vi "8channels_LEEMAN_081413.vi"() -> ()   [LabVIEW 2012]
doc: "Cont(inuous) Acq(uire) & Chart (hw timed) demonstrates the hardware timed, non-buffered technique of data acquisition. The scan clock on the board controls acquisition timing. Acquired scans are read directly from the device's FIFO using AI Single Scan. \n\nThe acquisition is configured with no buffer, and the on-board scan clock started at the selected scan rate. In the first loop iteration, the newest (most recent) scan is read from the FIFO. In each subsequent loop iteration AI Single Scan is called to read the oldest scan from the FIFO. Then if a scan is missed because the acquisition does not keep up, an error message will be displayed, and the acquisition stopped. Each scan is plotted on the chart after it is read. \n\nA common reason to use non-buffered acquisition is that some kind of processing needs to be done for each data point. You will probably want to add more functions to the diagram to customize this VI for your application. The acquisition rate you can achieve depends on how much processing and display the VI must do. This VI calls a subVI named My Single-Scan Processing. Add whatever processing you need to this subVI, or replace it with one of your own. The data processing subVI also demonstrates how to use error clusters in your own subVIs, so they can be included in the error data flow chain.\n\nBefore running this VI, set the values of the controls on the front panel. Select Show Help Window from the Help menu to see a description of each control. If the values you select for all the controls are values you will usually use, select Make Current Values Default from the Operate menu and save the VI. Or, you may save individual control's default values by popping up on the control, selecting Data Operations, then selecting Make Current Value Default, and saving the VI."
uses:
  <vilib>/DAQmx/read.llb/DAQmx Read (Analog 2D DBL NChan NSamp).vi
  BiaxGlobals.vi
  <vilib>/DAQmx/create/channels.llb/DAQmx Create Channel (AI-Voltage-Basic).vi
  <vilib>/DAQmx/configure/timing.llb/DAQmx Timing (Sample Clock).vi
  <vilib>/DAQmx/miscellaneous.llb/DAQmx Fill In Error Info.vi
panel:
  out "element 11":string
  out "element 10":string
  out "element 9":string
  out "element 8":string
  out "element 7":string
  out "element 6":string
  out "element 5":string
  out "element 4":string
  out "element 3":string
  out "element 2":string
  out "element":string
  out "element":string
  out "Stress-strain-temp vs time (Voltage)":dbl[][](graph)
  out "Array 13":i32[][](array[numeric])
  out "Array 12":i32[][](array[numeric])
  out "AUX8 (ch11)":dbl format="%.4f"
  out "AUX7 (ch10)":dbl format="%.4f"
  out "Array 11":i32[][](array[numeric])
  out "Array 10":i32[][](array[numeric])
  out "AUX6 (ch9)":dbl format="%.4f"
  out "AUX5 (ch8)":dbl format="%.4f"
  out "Array 9":i32[][](array[numeric])
  out "Array 8":i32[][](array[numeric])
  out "Array 7":i32[][](array[numeric])
  out "Array 6":i32[][](array[numeric])
  out "Array 5":i32[][](array[numeric])
  out "Array 4":i32[][](array[numeric])
  out "Array 3":i32[][](array[numeric])
  out "Array 2":i32[][](array[numeric])
  out "Array":i32[][](array[numeric])
  out "AUX4 (ch7)":dbl format="%.4f"
  out "AUX3 (ch6)":dbl format="%.4f"
  out "AUX2 (ch5)":dbl format="%.4f"
  out "AUX1 (ch4)":dbl format="%.4f"
  out "10000":bool
  in  "10 kHz":bool
  out "Processor scan rate":i32
  out "Present sample number":i32
  in  "1 Hz":bool
  out "1":bool
  out "10":bool
  out "100":bool
  out "1000":bool
  in  "10 Hz":bool
  in  "100 Hz":bool
  in  "1000 Hz":bool
  out "Data Recording Rate":i32(slide) scale=1.0..10000.0
  out "Write interval":i32
  out "Write countdown":i32
  out "Time into data acq. (s)":i32
  out "Saved sample No.":i32
  out "Record rate (samp/s)":i32
  out "No. of scans in backlog":i32
  out "Vert LVDT (ch3)":dbl format="%.4f"
  out "Vert Load (ch2)":dbl format="%.4f"
  out "Hor Load (ch0)":dbl format="%.4f"
  out "Hor LVDT (ch1)":dbl format="%.4f"
  in  "stop":bool
  # "Input Signals (volts)"
  # "To File (32 bit)"
  # "S\nI\nG\nN\nA\nL\n\nV\nO\nL\nT\nA\nG\nE"
  # "Timestamp"
  # "Acquisition Statistics"
  # "Data Recording Info"
  # "Sample (point) Number"
  # "NOTE:  This instrument will write data (time channel then Channels 0-3) to a user defined filename.  The file is written in binary format without a header.  \n            The time channel is comprised of numbers indicating the data recording frequency (eg 1, 10, 100, 1000, 10000  samples per second)."
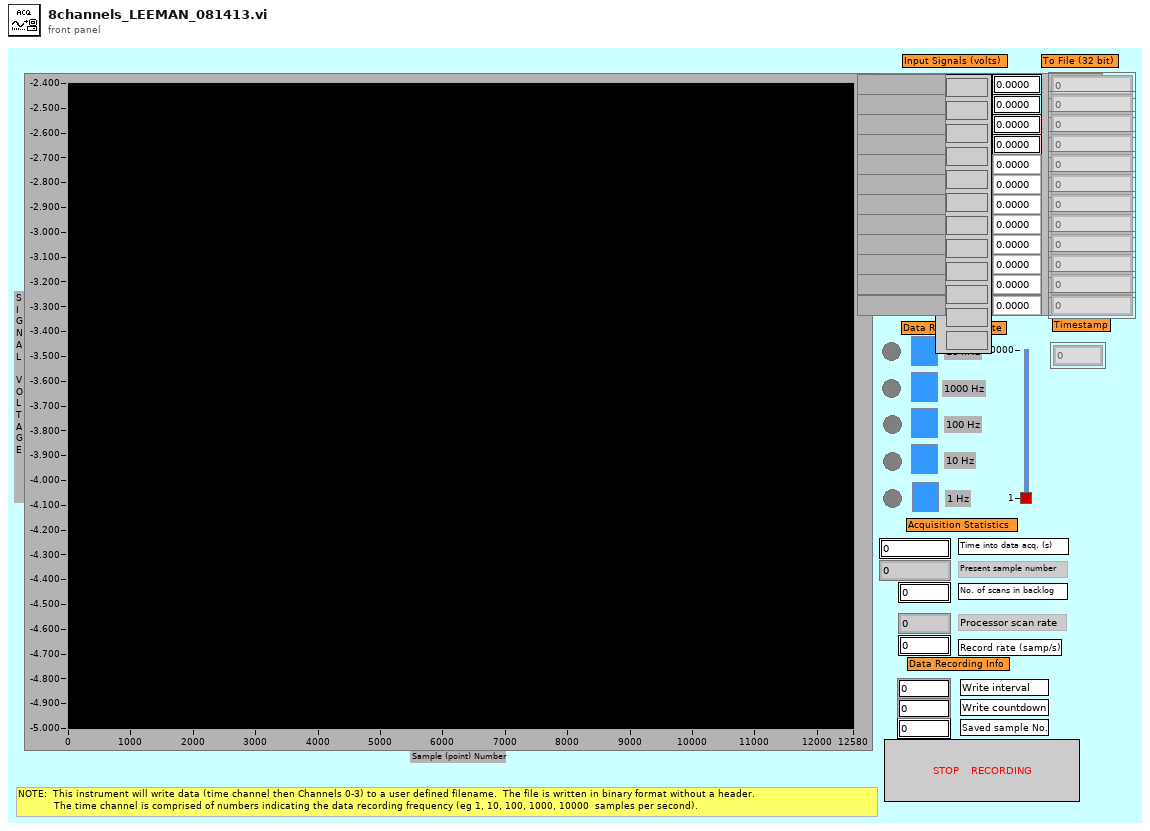
[diagram p1: front panel]
types:
  T1 = enum16{"big-endian, network order", "native, host order", "little-endian"}
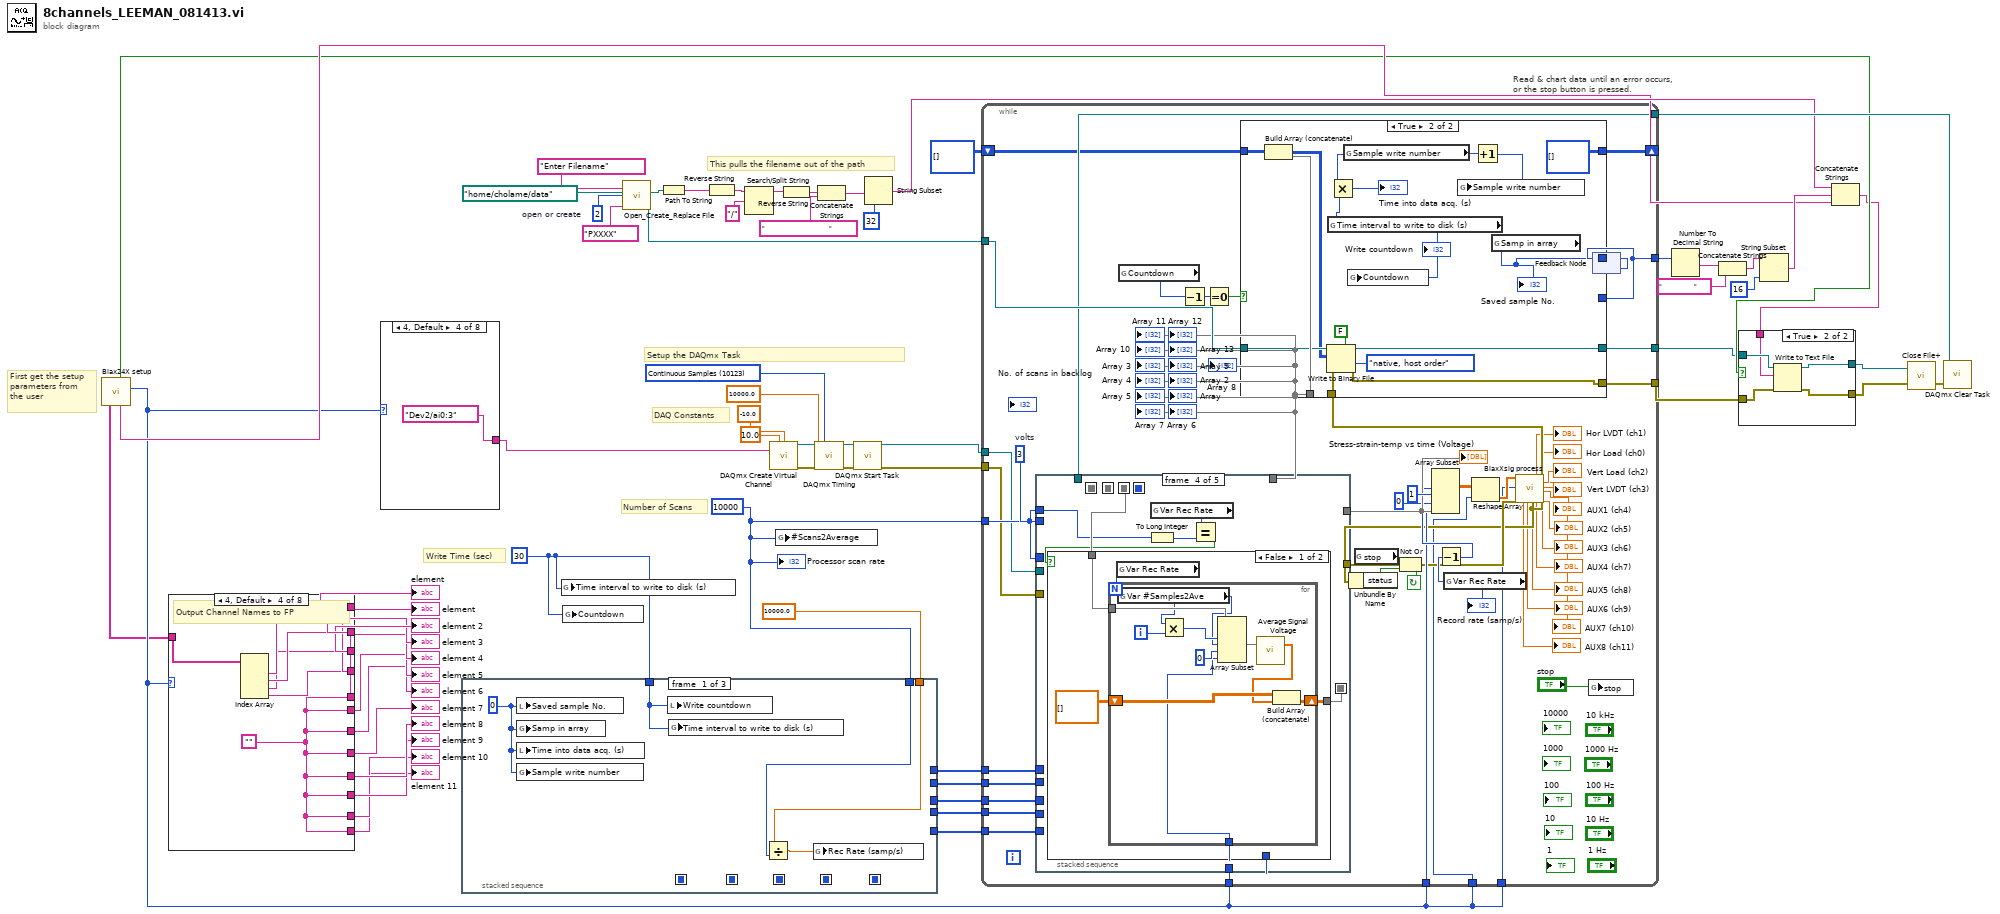
[diagram p0: block diagram]
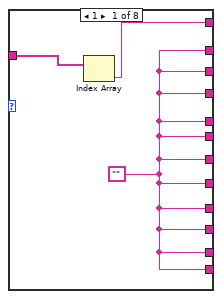
[diagram p2: hidden frame]
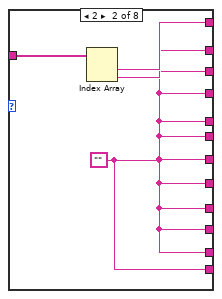
[diagram p3: hidden frame]
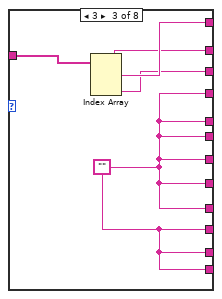
[diagram p4: hidden frame]
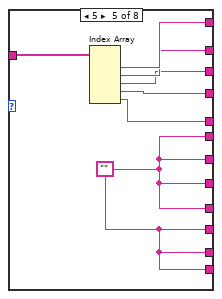
[diagram p5: hidden frame]
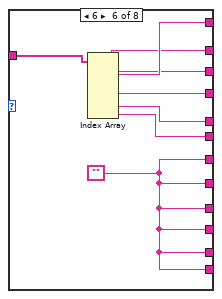
[diagram p6: hidden frame]
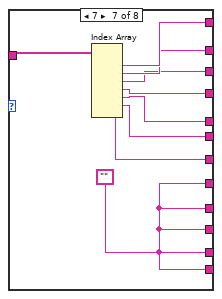
[diagram p7: hidden frame]
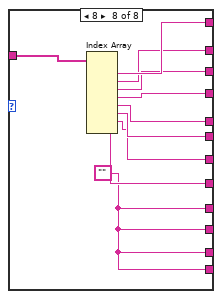
[diagram p8: hidden frame]
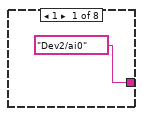
[diagram p10: hidden frame]
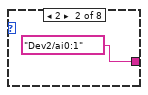
[diagram p11: hidden frame]
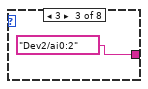
[diagram p12: hidden frame]
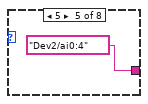
[diagram p13: hidden frame]
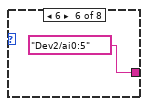
[diagram p14: hidden frame]
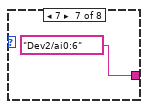
[diagram p15: hidden frame]
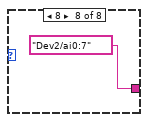
[diagram p16: hidden frame]
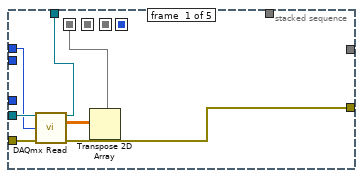
[diagram p17: hidden frame]
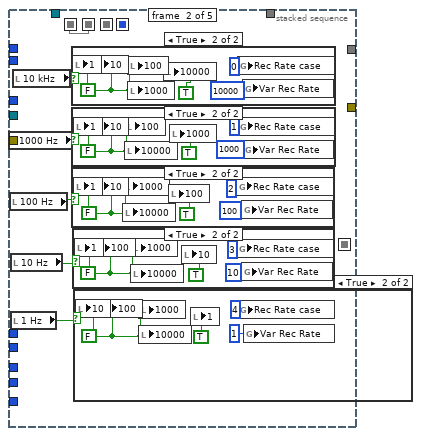
[diagram p18: hidden frame]
diagram:
  w6 = 10000 ("Number of scans")
  w7 = 30 ("Write time int (s)")
  w48 = 10123 items=["Finite Samples"=10178, "Continuous Samples"=10123, "Hardware Timed Single Point"=12522] ("sample mode")
  w64 = 2  # open or create
  # "Number of Scans"
  # "Write Time (sec)"
  # "First get the setup\nparameters from\nthe user"
  # "Setup the DAQmx Task"
  # "DAQ Constants"
  # "This pulls the filename out of the path"
  n1 = call "Biax24X setup.vi"() -> ("Footer String"=w29:string, "Number of Channels"=w22:i32, "ASCII footer 2"=w28:bool, "Channel Names"=w21:string[])  [unwired: 1 in, 4 out]
  n2 = case shown="4, Default" w22 {
    tunnel: w21 -> [w66 w70 w75 w81 w88 w96 w105 w116]
    tunnel: [w65 w71 w76 w82 w89 w97 w106 w115] -> w20
    tunnel: [w67 w69 w74 w80 w87 w95 w104 w114] -> w19
    tunnel: [w67 w68 w73 w79 w86 w94 w103 w113] -> w18
    tunnel: [w67 w68 w72 w78 w85 w93 w102 w112] -> w17
    tunnel: [w67 w68 w72 w77 w84 w92 w101 w111] -> w16
    tunnel: [w67 w68 w72 w77 w83 w91 w100 w110] -> w15
    tunnel: [w67 w68 w72 w77 w83 w90 w99 w109] -> w14
    tunnel: [w67 w68 w72 w77 w83 w90 w98 w108] -> w13
    tunnel: [w67 w68 w72 w77 w83 w90 w98 w107] -> w12
    tunnel: [w67 w68 w72 w77 w83 w90 w98 w107] -> w11
    tunnel: [w67 w68 w72 w77 w83 w90 w98 w107] -> w10
    tunnel: [w67 w68 w72 w77 w83 w90 w98 w107] -> w9
    frame 1 {
      w67 = ""
      n3 = Index Array(array=w66) -> (element=w65:string)  [unwired: 1 in]
    }
    frame 2 {
      w68 = ""
      n4 = Index Array(array=w70) -> (element #1=w71:string, element #2=w69:string)  [unwired: 2 in]
    }
    frame 3 {
      w72 = ""
      n5 = Index Array(array=w75) -> (element #1=w76:string, element #2=w74:string, element #3=w73:string)  [unwired: 3 in]
    }
    frame 4, Default {
      w77 = ""
      # "Output Channel Names to FP"
      n6 = Index Array(array=w81) -> (element #1=w82:string, element #2=w80:string, element #3=w79:string, element #4=w78:string)  [unwired: 4 in]
    }
    frame 5 {
      w83 = ""
      n7 = Index Array(array=w88) -> (element #1=w89:string, element #2=w87:string, element #3=w86:string, element #4=w85:string, element #5=w84:string)  [unwired: 5 in]
    }
    frame 6 {
      w90 = ""
      n8 = Index Array(array=w96) -> (element #1=w97:string, element #2=w95:string, element #3=w94:string, element #4=w93:string, element #5=w92:string, element #6=w91:string)  [unwired: 6 in]
    }
    frame 7 {
      w98 = ""
      n9 = Index Array(array=w105) -> (element #1=w106:string, element #2=w104:string, element #3=w103:string, element #4=w102:string, element #5=w101:string, element #6=w100:string, element #7=w99:string)  [unwired: 7 in]
    }
    frame 8 {
      w107 = ""
      n10 = Index Array(array=w116) -> (element #1=w115:string, element #2=w114:string, element #3=w113:string, element #4=w112:string, element #5=w111:string, element #6=w110:string, element #7=w109:string, element #8=w108:string)  [unwired: 8 in]
    }
  }
  "element" <- w20
  "element" <- w19
  "element 2" <- w18
  "element 3" <- w17
  "element 4" <- w16
  "element 5" <- w15
  "element 6" <- w14
  "element 7" <- w13
  "element 8" <- w12
  "element 9" <- w11
  "element 10" <- w10
  "element 11" <- w9
  n11 = case shown="4, Default" w22 {
    tunnel: [tag "Dev2/ai0" ("physical channels") tag "Dev2/ai0:1" ("physical channels") tag "Dev2/ai0:2" ("physical channels") tag "Dev2/ai0:3" ("physical channels") tag "Dev2/ai0:4" ("physical channels") tag "Dev2/ai0:5" ("physical channels") tag "Dev2/ai0:6" ("physical channels") tag "Dev2/ai0:7" ("physical channels")] -> w37
    frame 1 {
    }
    frame 2 {
    }
    frame 3 {
    }
    frame 4, Default {
    }
    frame 5 {
    }
    frame 6 {
    }
    frame 7 {
    }
    frame 8 {
    }
  }
  n12 = stacked-sequence {
    seq-local: [_ w145 _] -> [_ _ w158]
    seq-local: [_ w142 _] -> [_ _ w155]
    seq-local: [_ w137 _] -> [_ _ w157]
    seq-local: [_ w136 _] -> [_ _ w156]
    seq-local: [_ w131 _] -> [_ _ w154]
    tunnel: w7 -> [w126 _ _]
    tunnel: w6 -> [w129 _ _]
    tunnel: sgl 10000.0 ("actual scan rate") -> [w127 _ _]
    tunnel: [_ _ w158] -> w5
    tunnel: [_ _ w155] -> w4
    tunnel: [_ _ w157] -> w3
    tunnel: [_ _ w156] -> w2
    tunnel: [_ _ w154] -> w1
    frame #0 {
      w125 = i16 0
      n13 = local write "Saved sample No."(w125) -> ()
      n14 = global write "BiaxGlobals.vi" "Samp in array"(w125) -> ()
      n15 = local write "Time into data acq. (s)"(w125) -> ()
      n16 = global write "BiaxGlobals.vi" "Sample write number"(w125) -> ()
      n17 = local write "Write countdown"(w126) -> ()
      n18 = global write "BiaxGlobals.vi" "Time interval to write to disk (s)"(w126) -> ()
      n19 = Divide(x=w127, y=w129) -> (x/y=w128:sgl)
      n20 = global write "BiaxGlobals.vi" "Rec Rate (samp/s)"(w128) -> ()
    }
    frame #1 {
      n21 = local write "1"(TRUE) -> ()
      n22 = local write "10"(FALSE) -> ()
      n23 = local write "100"(FALSE) -> ()
      n24 = local write "1000"(FALSE) -> ()
      n25 = local write "10000"(FALSE) -> ()
      n26 = global read "BiaxGlobals.vi" "Time interval to write to disk (s)"() -> (→"Write interval":i32)
      n27 = global write "BiaxGlobals.vi" "Rec Rate case"(4) -> ()
      n28 = Initialize Array(i16 1, 10000) -> (w145:i16[])
      n29 = Initialize Array(i16 10, 1000) -> (w142:i16[])
      n30 = Initialize Array(i16 100, 100) -> (w137:i16[])
      n31 = Initialize Array(i16 1000, 10) -> (w136:i16[])
      n32 = Initialize Array(i16 10000, 1) -> (w131:i16[])
      n33 = global write "BiaxGlobals.vi" "Accum Time"(0) -> ()
      n34 = global write "BiaxGlobals.vi" "Var Rec Rate"(1) -> ()
    }
    frame #2 {
    }
  }
  n35 = global write "BiaxGlobals.vi" "Time interval to write to disk (s)"(w7) -> ()
  n36 = global write "BiaxGlobals.vi" "Countdown"(w7) -> ()
  n37 = call <vilib>:"Open_Create_Replace File.vi"("default name"="PXXXX", "prompt"="Enter Filename", "function (open:0)"=w64, "start path  (Not A Path)"=path "/home/cholame/data") -> ("new file path"=w59:path, "refnum"=w61:refnum<file>)  [unwired: 4 in, 2 out]
  n38 = Path To String(path=w59) -> (string=w56:string)
  n39 = Reverse String(1:w56) -> (0:w57:string)
  n40 = Search/Split String(string=w57, search string/char (-)="/") -> (substring before match=w55:string)  [unwired: 1 in, 2 out]
  n41 = call-poly <vilib>:"DAQmx Create Virtual Channel.vi"("maximum value"=10.0, "minimum value"=-10.0, "physical channels"=w37) -> ("task out"=w50:refnum<k21>, "error out"=w49:errorcluster)  [unwired: 11 in]
  n42 = global write "BiaxGlobals.vi" "#Scans2Average"(w6) -> ()
  n43 = Reverse String(1:w55) -> (0:w51:string)
  n44 = call-poly <vilib>:"DAQmx Timing.vi"("task/channels in"=w50, "sample mode"=w48, "rate"=10000.0, "error in"=w49) -> ("task out"=w47:refnum<k21>, "error out"=w46:errorcluster)  [unwired: 10 in]
  n45 = Concatenate Strings(w51, "                                ") -> (w53:string)
  n46 = call <vilib>:"DAQmx Start Task.vi"("task/channels in"=w47, "error in"=w46) -> ("task out"=w43:refnum<k21>, "error out"=w44:errorcluster)  [unwired: 12 in]
  n47 = String Subset(string=w53, length (rest)=32 ("length (rest)")) -> (substring=w30:string)  [unwired: 1 in]
  n48 = while "Read & chart data until an error occurs,\nor the stop button is pressed." {
    shift-left: i16[][] [] -> [w171]
    shift-right: [w205] -> _
    tunnel: w6 -> [w191]
    tunnel: [w206] -> w24
    tunnel: [w207] -> w27
    tunnel: w61 -> [w208]
    tunnel: w22 -> [w188]
    tunnel: w22 -> [w174]
    tunnel: w22 -> [w187]
    tunnel: w22 -> [w175]
    tunnel: w44 -> [w167]
    tunnel: w43 -> [w166]
    tunnel: [w199] -> w42
    tunnel: [w164] -> w36
    tunnel: w5 -> [w163]
    tunnel: w4 -> [w162]
    tunnel: w3 -> [w161]
    tunnel: w2 -> [w160]
    tunnel: w1 -> [w159]
    stop <- w204 continue-if-true
    w198 = 3  # volts
    n49 = stacked-sequence {
      seq-local: [w209 _ _ _ _] -> [_ w218 _ _ _]
      seq-local: [_ w218 _ _ _] -> [_ _ w244 _ _]
      seq-local: [_ _ w244 _ _] -> [_ _ _ w268 _]
      seq-local: [_ _ w243 _ _] -> [_ _ _ _ w294]
      seq-local: [_ _ _ w265 _] -> [_ _ _ _ w290]
      tunnel: [w215 _ _ _ _] -> w199
      tunnel: w198 -> [_ _ _ _ _]
      tunnel: w191 -> [w211 _ _ w267 _]
      tunnel: [w214 _ _ _ _] -> w185
      tunnel: [_ _ _ _ w290] -> w195
      tunnel: w191 -> [_ _ _ _ w293]
      tunnel: w163 -> [_ _ w254 _ _]
      tunnel: w162 -> [_ _ w253 _ _]
      tunnel: w161 -> [_ _ w252 _ _]
      tunnel: w160 -> [_ _ w251 _ _]
      tunnel: [_ _ _ _ w291] -> w168
      tunnel: w159 -> [_ _ w242 _ _]
      tunnel: w187 -> [_ _ _ w263 _]
      tunnel: w167 -> [w213 _ _ _ _]
      tunnel: w166 -> [w212 _ _ _ _]
      frame #0 {
        n50 = call-poly <vilib>:"DAQmx Read.vi"("task/channels in"=w212, "number of samples per channel"=w211, "error in"=w213) -> ("task out"=w215:refnum<k21>, "data"=w210:dbl[][], "error out"=w214:errorcluster)  [unwired: 10 in]
        n51 = Transpose 2D Array(2D array=w210) -> (transposed array=w209:dbl[][])
      }
      frame #1 {
        n52 = local read "1000 Hz"() -> (w221:bool)
        n53 = local read "100 Hz"() -> (w220:bool)
        n54 = local read "10 Hz"() -> (w219:bool)
        n55 = local read "1 Hz"() -> (w217:bool)
        n56 = local read "10 kHz"() -> (w216:bool)
        n57 = case shown="True" w216 {
          frame False {
          }
          frame True {
            w222 = FALSE
            n58 = local write "1"(w222) -> ()
            n59 = local write "10"(w222) -> ()
            n60 = local write "100"(w222) -> ()
            n61 = local write "1000"(w222) -> ()
            n62 = local write "10000"(TRUE ("10x")) -> ()
            n63 = global write "BiaxGlobals.vi" "Rec Rate case"(0) -> ()
            n64 = global write "BiaxGlobals.vi" "Var Rec Rate"(10000) -> ()
          }
        }
        n65 = case shown="True" w221 {
          frame False {
          }
          frame True {
            w238 = FALSE
            n66 = local write "1"(w238) -> ()
            n67 = local write "10"(w238) -> ()
            n68 = local write "100"(w238) -> ()
            n69 = local write "10000"(w238) -> ()
            n70 = local write "1000"(TRUE ("10x")) -> ()
            n71 = global write "BiaxGlobals.vi" "Rec Rate case"(1) -> ()
            n72 = global write "BiaxGlobals.vi" "Var Rec Rate"(1000) -> ()
          }
        }
        n73 = case shown="True" w220 {
          frame False {
          }
          frame True {
            w234 = FALSE
            n74 = local write "1"(w234) -> ()
            n75 = local write "10"(w234) -> ()
            n76 = local write "1000"(w234) -> ()
            n77 = local write "10000"(w234) -> ()
            n78 = local write "100"(TRUE ("1x")) -> ()
            n79 = global write "BiaxGlobals.vi" "Rec Rate case"(2) -> ()
            n80 = global write "BiaxGlobals.vi" "Var Rec Rate"(100) -> ()
          }
        }
        n81 = case shown="True" w219 {
          frame False {
          }
          frame True {
            w230 = FALSE
            n82 = local write "1"(w230) -> ()
            n83 = local write "100"(w230) -> ()
            n84 = local write "1000"(w230) -> ()
            n85 = local write "10000"(w230) -> ()
            n86 = local write "10"(TRUE ("0.1x")) -> ()
            n87 = global write "BiaxGlobals.vi" "Rec Rate case"(3) -> ()
            n88 = global write "BiaxGlobals.vi" "Var Rec Rate"(10) -> ()
          }
        }
        n89 = case shown="True" w217 {
          frame False {
          }
          frame True {
            w226 = FALSE
            n90 = local write "10"(w226) -> ()
            n91 = local write "100"(w226) -> ()
            n92 = local write "1000"(w226) -> ()
            n93 = local write "10000"(w226) -> ()
            n94 = local write "1"(TRUE) -> ()
            n95 = global write "BiaxGlobals.vi" "Rec Rate case"(4) -> ()
            n96 = global write "BiaxGlobals.vi" "Var Rec Rate"(1) -> ()
          }
        }
      }
      frame #2 {
        n97 = global read "BiaxGlobals.vi" "Rec Rate case"() -> (w250:i32)
        n98 = case shown="3" w250 {
          tunnel: w254 -> [w258 _ _ _ _]
          tunnel: [w258 w259 w260 w261 w262] -> w243
          tunnel: w253 -> [_ w259 _ _ _]
          tunnel: w252 -> [_ _ w260 _ _]
          tunnel: w251 -> [_ _ _ w261 _]
          tunnel: w242 -> [_ _ _ _ w262]
          frame ..0 {
          }
          frame 1 {
          }
          frame 2 {
          }
          frame 3 {
          }
          frame 4.. {
          }
        }
        n99 = Array Size(array=w243) -> (size(s)=w247:i32)
        n100 = global read "BiaxGlobals.vi" "Countdown"() -> (w246:i32)
        n101 = global read "BiaxGlobals.vi" "Samp in array"() -> (w249:i32)
        n102 = Add(x=w249, y=w247) -> (x+y=w248:i32)
        "Present sample number" <- w248
        n103 = global read "BiaxGlobals.vi" "Var Rec Rate"() -> (w256:i32)
        "Data Recording Rate" <- w256
        n104 = global write "BiaxGlobals.vi" "Samp in array"(w248) -> ()
        n105 = global read "BiaxGlobals.vi" "#Scans2Average"() -> (w257:i16)
        n106 = Divide(x=w257, y=w256) -> (x/y=w255:dbl)
        n107 = Decrement(x=w246) -> (x-1=w245:i32)
        n108 = global write "BiaxGlobals.vi" "Var #Samples2Ave"(w255) -> ()
        n109 = local write "Write countdown"(w245) -> ()
      }
      frame #3 {
        n110 = To Long Integer(number=w267) -> (32bit integer=w266:i32)
        n111 = global read "BiaxGlobals.vi" "Var Rec Rate"() -> (w269:i32)
        n112 = Equal?(x=w269, y=w266) -> (x = y?=w264:bool)
        n113 = case shown="False" w264 {
          tunnel: w268 -> [w273 w285]
          tunnel: [w272 w285] -> w265
          tunnel: w263 -> [w270 _]
          frame False {
            n114 = global read "BiaxGlobals.vi" "Var Rec Rate"() -> (w271:i32)
            n115 = for {
              N: w271 -> [_]
              shift-right: [w284] -> w272
              shift-left: dbl[][] [] -> [w280]
              tunnel: w273 -> [w283]
              tunnel: w270 -> [w277]
              i -> [w278]
              n116 = global read "BiaxGlobals.vi" "Var #Samples2Ave"() -> (w275:i32)
              n117 = Multiply(x=w275, y=w278) -> (x*y=w276:i32)
              n118 = Array Subset(array=w283, index (row)=w276, length (row)=w275, index (col)=i16 0, length (col)=w277) -> (w282:dbl[][])
              n119 = call "Average Signal Voltage.vi"("voltage data"=w282) -> ("average value\nper channel"=w279:dbl[])  [unwired: 2 in]
              n120 = Build Array (concatenate)(w280, w279) -> (w284:dbl[][])
            }
          }
          frame True {
          }
        }
      }
      frame #4 {
        (unwired) 1000.0
        n121 = global read "BiaxGlobals.vi" "Accum Time"() -> (w296:dbl)
        n122 = Transpose 2D Array(2D array=w290) -> (transposed array=w289:dbl[][])
        n123 = Multiply(x=838860.8, y=w289) -> (x*y=w287:dbl[][])
        n124 = To Long Integer(number=w287) -> (32bit integer=w286:i32[][])
        n125 = Add(x=w293, y=w296) -> (x+y=w295:dbl)
        n126 = Build Array (concatenate)(w294, w286) -> (w292:i32[][])
        n127 = global write "BiaxGlobals.vi" "Accum Time"(w295) -> ()
        n128 = Transpose 2D Array(2D array=w292) -> (transposed array=w291:i32[][])
      }
    }
    "Stress-strain-temp vs time (Voltage)" <- w195
    "Array" <- w168
    "Array 2" <- w168
    "Array 3" <- w168
    "Array 4" <- w168
    "Array 5" <- w168
    "Array 6" <- w168
    "Array 7" <- w168
    "Array 8" <- w168
    "Array 9" <- w168
    "Array 10" <- w168
    "Array 11" <- w168
    "Array 12" <- w168
    "Array 13" <- w168
    n129 = global read "BiaxGlobals.vi" "Countdown"() -> (w190:i32)
    n130 = Decrement(x=w190) -> (x-1=w189:i32)
    n131 = Equal To 0?(x=w189) -> (x = 0?=w200:bool)
    n132 = global read "BiaxGlobals.vi" "stop"() -> (w201:bool)
    n133 = global read "BiaxGlobals.vi" "Var Rec Rate"() -> (w193:i32)
    "Record rate (samp/s)" <- w193
    n134 = Decrement(x=w193) -> (x-1=w192:i32)
    n135 = Array Subset(array=w195, index (row)=w192, length (row)=1, index (col)=0, length (col)=w188) -> (w196:dbl[][])
    n136 = Reshape Array(w196, w174) -> (w186:dbl[])
    n137 = call "BiaxXsig process.vi"("voltage data"=w186, "Numeric"=w175, "error in (no error)"=w185) -> ("AUX8"=→"AUX8 (ch11)":dbl, "AUX7"=→"AUX7 (ch10)":dbl, "AUX6"=→"AUX6 (ch9)":dbl, "AUX5"=→"AUX5 (ch8)":dbl, "error out"=w184:errorcluster, "Hor LVDT"=→"Hor LVDT (ch1)":dbl, "AUX4"=→"AUX4 (ch7)":dbl, "Hor Load"=→"Hor Load (ch0)":dbl, "Vert Load"=→"Vert Load (ch2)":dbl, "Vert LVDT"=→"Vert LVDT (ch3)":dbl, "AUX1"=→"AUX1 (ch4)":dbl, "AUX2"=→"AUX2 (ch5)":dbl, "AUX3"=→"AUX3 (ch6)":dbl)  [unwired: 3 in, 1 out]
    n138 = Unbundle By Name(w184) -> ("status"=w203:bool)
    n139 = Not Or(1:w203, 2:w201) -> (0:w204:bool)
    n140 = global write "BiaxGlobals.vi" "stop"("stop") -> ()
    n141 = feedback #1() -> (w164:i32)  [unwired: 1 in]
    n142 = case shown="True" w200 {
      tunnel: w168 -> [w304 w314]
      tunnel: w171 -> [w303 w315]
      tunnel: w208 -> [w302 w311]
      tunnel: [w302 w310] -> w207
      tunnel: w184 -> [w301 w312]
      tunnel: [w301 w309] -> w206
      tunnel: [w298 i16[][] []] -> w205
      tunnel: [w297 w307] -> w165
      tunnel: w164 -> [w297 _]
      frame False {
        n143 = Build Array (concatenate)(w303, w304) -> (w298:i32[][])
        n144 = global read "BiaxGlobals.vi" "Countdown"() -> (w300:i32)
        n145 = Decrement(x=w300) -> (x-1=w299:i32)
        n146 = global write "BiaxGlobals.vi" "Countdown"(w299) -> ()
      }
      frame True {
        n147 = Build Array (concatenate)(w315, w314) -> (w308:i32[][])
        n148 = Write to Binary File(file (use dialog)=w311, data=w308, error in=w312, 5:FALSE ("prepend array or string size? (T)"), 9:T1."native, host order" ("byte order (0:big-endian, network order)")) -> (refnum out=w310:refnum<file>, error out=w309:errorcluster)  [unwired: 1 in, 1 out]
        n149 = global read "BiaxGlobals.vi" "Time interval to write to disk (s)"() -> (w316:i32)
        "Write countdown" <- w316
        n150 = global read "BiaxGlobals.vi" "Sample write number"() -> (w319:i16)
        n151 = global write "BiaxGlobals.vi" "Countdown"(w316) -> ()
        n152 = Increment(x=w319) -> (x+1=w313:i16)
        n153 = Multiply(x=w313, y=w316) -> (x*y=→"Time into data acq. (s)":i32)
        n154 = global write "BiaxGlobals.vi" "Sample write number"(w313) -> ()
        n155 = global read "BiaxGlobals.vi" "Samp in array"() -> (w307:i32)
        "Saved sample No." <- w307
      }
    }
    n156 = feedback-in #1(w165) -> ()
  }
  n157 = Number To Decimal String(number=w36) -> (decimal integer string=w35:string)  [unwired: 1 in]
  n158 = Concatenate Strings(w35, "                " ("string")) -> (w33:string)
  n159 = String Subset(string=w33, length (rest)=16 ("length (rest)")) -> (substring=w31:string)  [unwired: 1 in]
  n160 = Concatenate Strings(w30, w31, w29) -> (w23:string)
  n161 = case shown="True" w28 {
    tunnel: [w321 w325] -> w26
    tunnel: w27 -> [w321 w326]
    tunnel: w24 -> [w320 w323]
    tunnel: [w320 w324] -> w25
    tunnel: w23 -> [_ w322]
    frame False {
    }
    frame True {
      n162 = Write to Text File(file (use dialog)=w326, text=w322, error in=w323) -> (refnum out=w325:refnum<file>, error out=w324:errorcluster)  [unwired: 1 in, 1 out]
    }
  }
  n163 = call "Close File+.vi"("error in (no error)"=w25, "refnum"=w26) -> ("error out"=w45:errorcluster)  [unwired: 3 in, 2 out]
  n164 = call <vilib>:"DAQmx Clear Task.vi"("task in"=w42, "error in"=w45) -> ()  [unwired: 13 in, 1 out]
  "Processor scan rate" <- w6
